vi "Configure Multi Eval Meas EVM Offset Limit.vi"(5 "Peak":dbl[](array[numeric]) format="%^.3e", 6 "Peak Enabled":bool[](array[boolean]), 7 "RMS":dbl[](array[numeric]) format="%^.3e", 8 "error in (no error)":errorcluster, 9 "RMS Enabled":bool[](array[boolean]), 10 "Instance (1)":i32=1, 11 "VISA resource name":refnum<visa-resource-name>) -> (0 "error out":errorcluster, 3 "VISA resource name out":refnum<visa-resource-name>)   [LabVIEW 2015, in "Rohde&Schwarz CMP LR WPAN Measurement.lvlib"]
doc: "Defines upper limits for the RMS and peak values of the offset error vector magnitude (EVM).\n\nOrder of parameters:\n<1_RMS_EVM_PS> - RMS offset EVM for PSDU portion\n<2_Peak_EVM_PS> - Peak offset EVM for PSDU portion\n<3_RMS_PS_Enb> - Disables | enables the limit check for RMS offset EVM within PSDU portion.\n<4_Peak_PS_Enb> - Disables | enables the limit check for peak offset EVM within PSDU portion.\n<5_RMS_EVM_SP> - RMS offset EVM for SHR + PHR portion\n<6_Peak_EVM_SP> - Peak offset EVM for SHR + PHR portion\n<7_RMS_EVM_All> - Overall RMS offset EVM for complete PPDU\n<8_Peak_EVM_All> - Overall Peak offset EVM for complete PPDU\n<9_RMS_SP_Enb> - Disables | enables the RMS limit check for offset EVM within SHR + PHR portion.\n<10_Peak_SP_Enb> - Disables | enables the peak limit check for offset EVM within SHR + PHR portion.\n<11_RMS_Sll_Enb> - Disables | enables the RMS limit check for overall offset EVM for complete PPDU.\n<12_Peak_All_Enb> - Disables | enables the peak limit check for overall offset EVM for complete PPDU.\n\nAttribute:\n-\n\nRemote-control command:\nCONFigure:WPAN:MEAS<i>:MEValuation:LIMit:EVM[:OFFSet]"
uses:
  <instrlib>/Rohde&Schwarz CMP LR WPAN Measurement/Rohde&Schwarz CMP LR WPAN Measurement.lvlib
  <instrlib>/Rohde&Schwarz CMP LR WPAN Measurement/Private/rsidr_core.llb/rsidr_core.lvlib
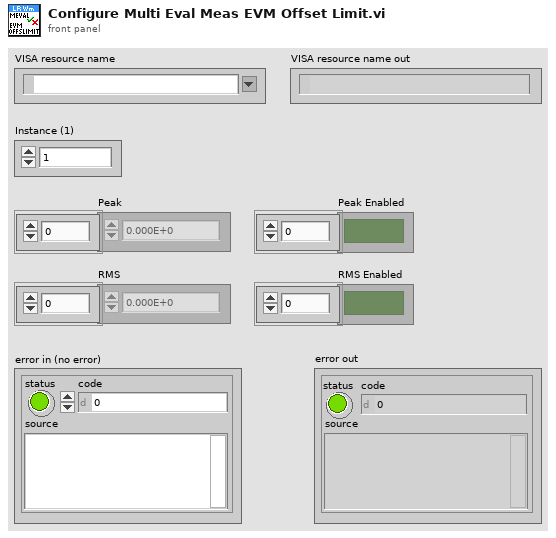
[diagram p1: front panel]
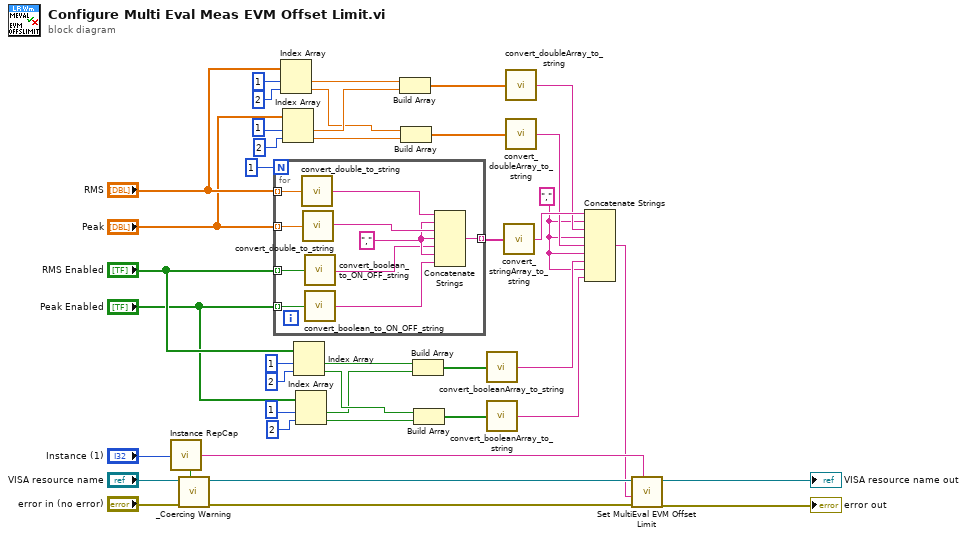
[diagram p0: block diagram]
diagram:
  w2 = "," ("string")
  n1 = call <instrlib>:"Instance RepCap.vi"("Instance In"="Instance (1)") -> ("In Range?"=w41:bool, "RepCap Identifier Out"=w40:string)  [unwired: 1 in]
  n2 = call <instrlib>:"_Coercing Warning.vi"("In Range?"=w41, "error in (no error)"="error in (no error)", "VISA resource name"="VISA resource name") -> ("error out"=w37:errorcluster, "VISA resource name out"=w36:refnum<visa-resource-name>)  [unwired: 7 in]
  n3 = for {
    N: 1 -> [_]
    tunnel: "RMS" -> [w50] mode=indexing
    tunnel: "Peak" -> [w49] mode=indexing
    tunnel: "RMS Enabled" -> [w52] mode=indexing
    tunnel: "Peak Enabled" -> [w51] mode=indexing
    tunnel: [w47] -> w33 mode=indexing
    w44 = "," ("string")
    n4 = call <instrlib>:"convert_double_to_string.vi"("double in"=w50) -> ("string out"=w48:string)  [unwired: 4 in]
    n5 = call <instrlib>:"convert_double_to_string.vi"("double in"=w49) -> ("string out"=w46:string)  [unwired: 4 in]
    n6 = call <instrlib>:"convert_boolean_to_ON_OFF_string.vi"("boolean value in"=w52) -> ("string value out"=w43:string)  [unwired: 4 in]
    n7 = call <instrlib>:"convert_boolean_to_ON_OFF_string.vi"("boolean value in"=w51) -> ("string value out"=w45:string)  [unwired: 4 in]
    n8 = Concatenate Strings(w48, w44, w46, w44, w43, w44, w45) -> (w47:string)
  }
  n9 = Index Array(array="RMS", index #1=1, index #2=2) -> (element #1=w25:dbl, element #2=w24:dbl)
  n10 = Index Array(array="Peak", index #1=1, index #2=2) -> (element #1=w26:dbl, element #2=w23:dbl)
  n11 = Index Array(array="RMS Enabled", index #1=1, index #2=2) -> (element #1=w15:bool, element #2=w14:bool)
  n12 = Index Array(array="Peak Enabled", index #1=1, index #2=2) -> (element #1=w12:bool, element #2=w13:bool)
  n13 = Build Array(w25, w26) -> (w22:dbl[])
  n14 = Build Array(w24, w23) -> (w21:dbl[])
  n15 = Build Array(w15, w12) -> (w10:bool[])
  n16 = Build Array(w14, w13) -> (w9:bool[])
  n17 = call <instrlib>:"convert_booleanArray_to_string.vi"("Boolean array in"=w10) -> ("string out"=w11:string)  [unwired: 4 in]
  n18 = call <instrlib>:"convert_booleanArray_to_string.vi"("Boolean array in"=w9) -> ("string out"=w8:string)  [unwired: 4 in]
  n19 = call <instrlib>:"convert_stringArray_to_string.vi"("string array in"=w33) -> ("string out"=w32:string)  [unwired: 4 in]
  n20 = call <instrlib>:"convert_doubleArray_to_string.vi"("double array in"=w22) -> ("string out"=w31:string)  [unwired: 4 in]
  n21 = call <instrlib>:"convert_doubleArray_to_string.vi"("double array in"=w21) -> ("string out"=w20:string)  [unwired: 4 in]
  n22 = Concatenate Strings(w32, w2, w31, w2, w20, w2, w11, w2, w8) -> (w7:string)
  n23 = call "Set MultiEval EVM Offset Limit"("Repeated Capabilities"=w40, "error in (no error)"=w37, "MultiEval EVM Offset Limit ()"=w7, "instrument handle"=w36) -> ("error out"=→"error out":errorcluster, "instrument handle out"=→"VISA resource name out":refnum<visa-resource-name>)  [unwired: 6 in]
